vi "Reduce Title length.vi"(3 "Reduce Individual Plot Title Lengths if too long":bool=TRUE, 4 "Array in":string[](array[string]), 5 "No of Charcters":i32=20) -> (1 "Array out":string[](array[string]))   [LabVIEW 2022 SP3]
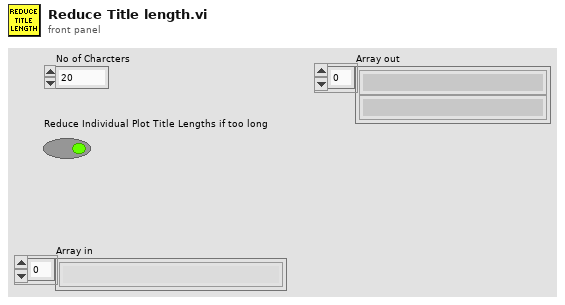
[diagram p1: front panel]
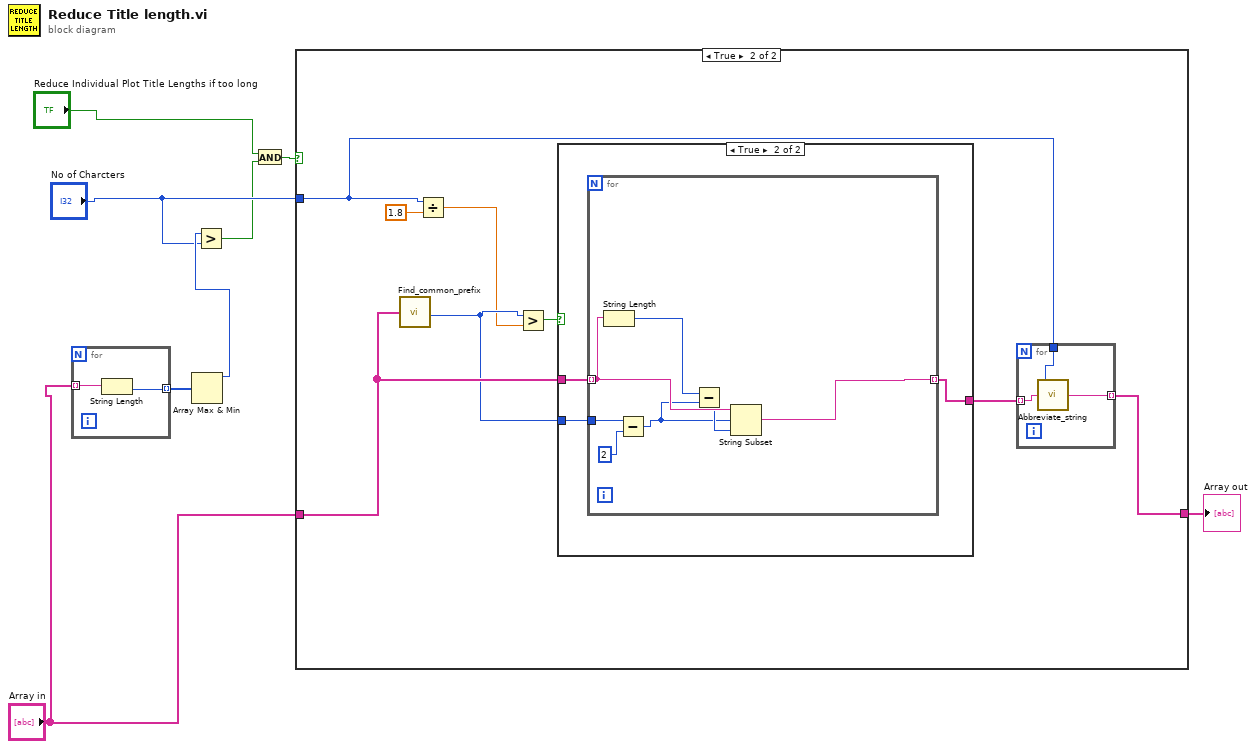
[diagram p0: block diagram]
diagram:
  n1 = for {
    tunnel: "Array in" -> [w10] mode=indexing
    tunnel: [w9] -> w6 mode=indexing
    n2 = String Length(string=w10) -> (length=w9:i32)
  }
  n3 = Array Max & Min(array=w6) -> (max value=w5:i32)  [unwired: 3 out]
  n4 = Greater?(x=w5, y="No of Charcters") -> (0:w2:bool)
  n5 = And(x="Reduce Individual Plot Title Lengths if too long", y=w2) -> (x .and. y?=w3:bool)
  n6 = case shown="True" w3 {
    tunnel: "Array in" -> [w11 w19]
    tunnel: [w11 w15] -> w8
    tunnel: "No of Charcters" -> [_ w12]
    frame False {
    }
    frame True {
      n7 = call "Find_common_prefix.vi"("Input Array"=w19) -> ("Common Characters"=w17:i32)
      n8 = Divide(x=w12, y=1.8) -> (x/y=w13:dbl)
      n9 = Greater?(x=w17, y=w13) -> (0:w18:bool)
      n10 = case shown="True" w18 {
        tunnel: w19 -> [w23 w26]
        tunnel: w17 -> [_ w25]
        tunnel: [w23 w24] -> w16
        frame False {
        }
        frame True {
          n11 = for {
            tunnel: [w30] -> w24 mode=indexing
            tunnel: w26 -> [w33] mode=indexing
            tunnel: w25 -> [w29]
            n12 = String Length(string=w33) -> (length=w32:i32)
            n13 = Subtract(x=w29, y=2) -> (x-y=w27:i32)
            n14 = Subtract(x=w32, y=w27) -> (x-y=w31:i32)
            n15 = String Subset(string=w33, offset (0)=w27, length (rest)=w31) -> (substring=w30:string)
          }
        }
      }
      n16 = for {
        tunnel: w16 -> [w22] mode=indexing
        tunnel: [w21] -> w15 mode=indexing
        tunnel: w12 -> [w20]
        n17 = call "Abbreviate_string.vi"("Input String"=w22, "Max String Length"=w20) -> ("Output String"=w21:string)  [unwired: 1 in, 2 out]
      }
    }
  }
  "Array out" <- w8
